vi "Replace Values Array Multiple Timestamps.vi"(4 "Values (new)":u8[](array[numeric]), 6 "Timestamps (new)":u64[](array[numeric]), 7 "#bytes per timestamp":i32, 9 "index":i32, 10 "Values (buffered)":u8[](array[numeric]), 11 "Timestamps (buffered)":u64[](array[numeric])) -> (2 "Values (buffered)":u8[](array[numeric]), 3 "Timestamps (buffered)":u64[](array[numeric]))   [LabVIEW 2021, in "Ring Buffer Time Series Data.lvlib"]
uses:
  Ring Buffer Time Series Data.lvlib
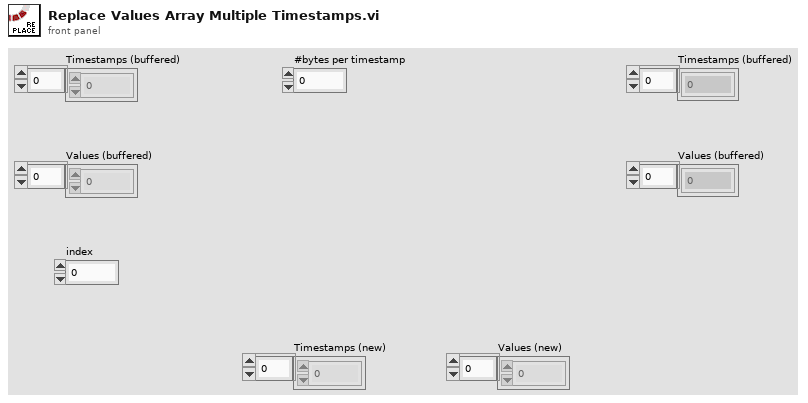
[diagram p1: front panel]
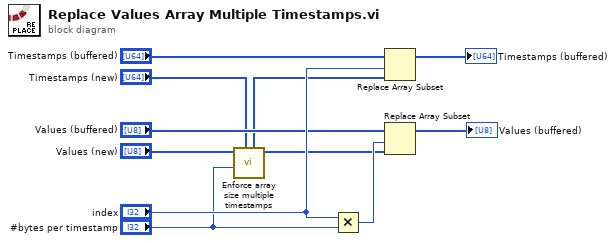
[diagram p0: block diagram]
diagram:
  n1 = call "Enforce array size multiple timestamps.vi"("Timestamps (new)"="Timestamps (new)", "#bytes per timestamp"="#bytes per timestamp", "Values (new)"="Values (new)") -> ("Values (new) [padded]"=w1:u8[], "Timestamps (new)"=w2:u64[])  [unwired: 7 in]
  n2 = Multiply(x="index", y="#bytes per timestamp") -> (x*y=w7:i32)
  n3 = Replace Array Subset(array="Timestamps (buffered)", new element=w2, index="index") -> (→"Timestamps (buffered)":u64[])
  n4 = Replace Array Subset(array="Values (buffered)", new element=w1, index=w7) -> (→"Values (buffered)":u8[])
